vi "chart axis set minor unit.vi"(8 "error in (no error)":errorcluster, 10 "unit":dbl, 11 "axis":u32) -> (0 "error out":errorcluster)   [LabVIEW 2015, in "xlsxwriter.lvlib"]
doc: "void chart_axis_set_minor_unit(lxw_chart_axis axis, double unit);"
uses:
  xlsxwriter.lvlib
  xlsxwriter.dll
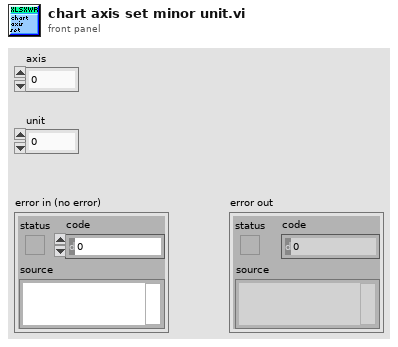
[diagram p1: front panel]
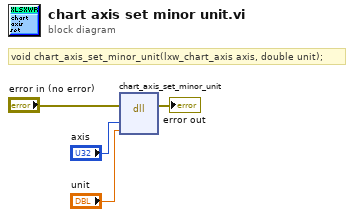
[diagram p0: block diagram]
diagram:
  # "void chart_axis_set_minor_unit(lxw_chart_axis axis, double unit);"
  n1 = dll-call lib="C:/Users/WDAGUtilityAccount/Desktop/lv_vis_added_cell/xlsxwriter.*" fn="chart_axis_set_minor_unit"(error in="error in (no error)", "axis"="axis", "unit"="unit") -> (error out=→"error out":errorcluster)  [unwired: 5 in, 1 out]
